vi "Insert Key Value Pair (Boolean Array).vi"(7 "key":string, 8 "error in (no error)":errorcluster, 10 "JSON Data in":bool[](array[boolean]), 11 "JSON Object in":refnum<class "JSON Helper.lvclass">) -> (0 "error out":errorcluster, 1 "replaced":bool, 3 "JSON Object Out":refnum<class "JSON Helper.lvclass">)   [LabVIEW 2016, in "JSON Helper.lvclass"]
uses:
  JSON Helper/JSON Helper.lvclass
  JSON Array/New JSON Array (Boolean).vi
  Insert Key Value Pair (Single String).vi
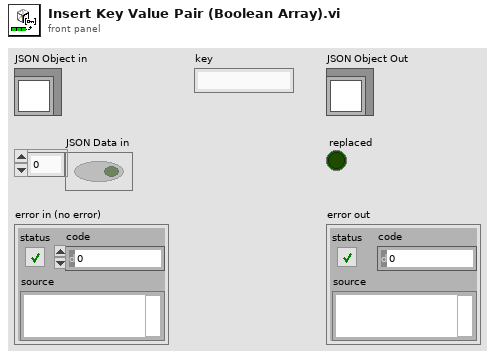
[diagram p1: front panel]
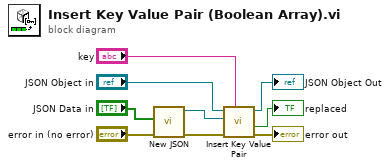
[diagram p0: block diagram]
diagram:
  n1 = call-poly "New JSON.vi"("error in (no error)"="error in (no error)", "Boolean Array"="JSON Data in") -> ("error out"=w8:errorcluster, "JSON Array out"=w9:refnum<class "JSON Helper.lvclass">)  [unwired: 8 in]
  n2 = call-poly "Insert Key Value Pair.vi"("key"="key", "error in (no error)"=w8, "value"=w9, "JSON Object in"="JSON Object in") -> ("error out"=→"error out":errorcluster, "replaced"=→"replaced":bool, "JSON Object out"=→"JSON Object Out":refnum<class "JSON Helper.lvclass">)  [unwired: 5 in]
